vi "CSM - Forward UI Operations to CSM.vi"(7 "Name(\"\" to use uuid)":string, 11 "State(s) in (\"\")":string) -> (3 "States Out":string)   [LabVIEW 2020, in "Communicable State Machine.lvlib"]
uses:
  Communicable State Machine.lvlib
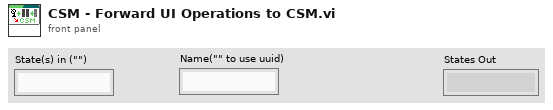
[diagram p1: front panel]
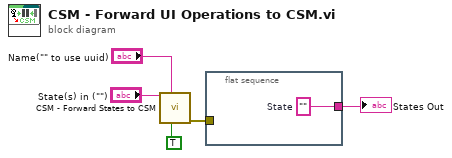
[diagram p0: block diagram]
diagram:
  n1 = call "CSM - Forward States to CSM.vi"("High Priority(T)"=TRUE, "Module Name"="Name(\"\" to use uuid)", "State(s) in (\"\")"="State(s) in (\"\")") -> ("error out"=w1:errorcluster)  [unwired: 8 in]
  n2 = flat-sequence {
    tunnel: [w6] -> w5
    tunnel: w1 -> [_]
    frame #0 {
      w6 = ""  # State
    }
  }
  "States Out" <- w5
